vi "Public.vi"() -> ()   [LabVIEW 2015, in "Circle.lvclass"]
uses:
  Circle.lvclass
  colors.ctl
  Circle.lvclass/Circle.ctl
panel:
  out "output cluster":refnum<class "Circle.lvclass">
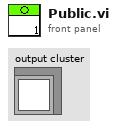
[diagram p1: front panel]
types:
  T1 = typedef "colors.ctl" = enum16{"Blue", "Red", "Green", "Yellow"}
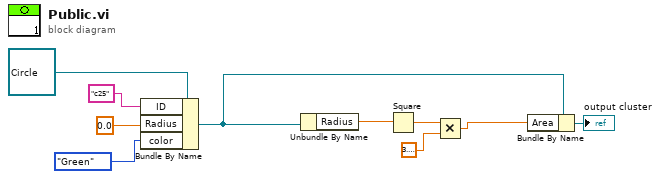
[diagram p0: block diagram]
diagram:
  n1 = Bundle By Name(cluster=refnum<class "Circle.lvclass"> refnum ("Circle.lvclass"), "ID"="c25", "Radius"=0.0, "color"=colors."Green") -> (w6:refnum<class "Circle.lvclass">)
  n2 = Unbundle By Name(w6) -> ("Radius"=w9:dbl)
  n3 = Square(x=w9) -> (x^2=w8:dbl)
  n4 = Multiply(x=w8, y=3.141592653589793) -> (x*y=w5:dbl)
  n5 = Bundle By Name(cluster=w6, "Area"=w5) -> (→"output cluster":refnum<class "Circle.lvclass">)
